vi "Maximize.vi"(8 "error in":errorcluster, 11 "Philips Dialog in":refnum<class "Flex UI Dialog.lvclass">) -> (0 "error out":errorcluster, 3 "Philips Dialog out":refnum<class "Flex UI Dialog.lvclass">)   [LabVIEW 2014, in "Flex UI Dialog.lvclass"]
doc: "Maximizes the UI."
uses:
  Flex UI Dialog.lvclass
  Flex UI (Parent)/Flex UI.lvclass/Flex UI.ctl
  Flex UI (Parent)/Flex UI.lvclass
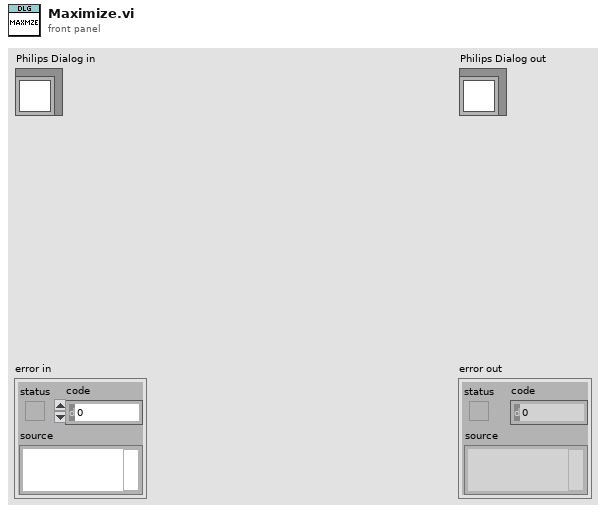
[diagram p1: front panel]
types:
  T1 = enum32{"Invalid", "Standard", "Closed", "Hidden", "Minimized", "Maximized"}
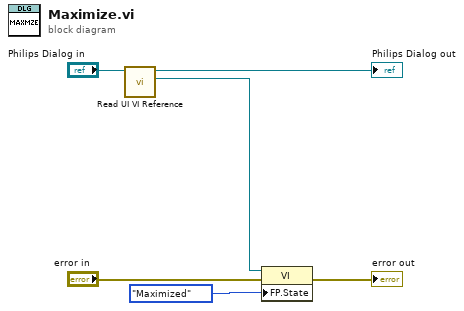
[diagram p0: block diagram]
diagram:
  n1 = call "Read UI VI Reference.vi"("Philips UI in"="Philips Dialog in") -> ("UI VI Reference"=w2:refnum<vi>, "Philips UI out"=→"Philips Dialog out":refnum<class "Flex UI Dialog.lvclass">)  [unwired: 9 in]
  n2 = property class="VI"(reference=w2, error in="error in", "FP.State"=T1."Maximized" ("Front Panel Window:State")) -> (error out=→"error out":errorcluster)  [unwired: 1 out]
